vi "insert_spirals.vi"(8 "error in (no error)":errorcluster, 9 "angular shift":dbl, 10 "SpaceVector in":refnum<class "SpaceVector.lvclass">, 11 "TrajectoryDL121017Hopping in":refnum<class "TrajectoryDL121017Hopping.lvclass">) -> (0 "error out":errorcluster, 2 "fix point with spirals":refnum<class "SpaceVector.lvclass">[](array[class]), 3 "TrajectoryDL121017Hopping out":refnum<class "TrajectoryDL121017Hopping.lvclass">)   [LabVIEW 2010, in "TrajectoryDL121017Hopping.lvclass"]
uses:
  TrajectoryDL121017Hopping.lvclass
  common/classes/SpaceVector/SpaceVector/SpaceVector.lvclass
  <vilib>/Native 3D Graph/xcontrol/3DPC_SurfacePlot.xctl
  TrajectoryDL121017Hopping.lvclass/TrajectoryDL121017Hopping.ctl
panel:
  out "3D Graph 2":refnum<class "Base Datatype.lvclass">[](xcontrol)
  in  "number of points":i32=100
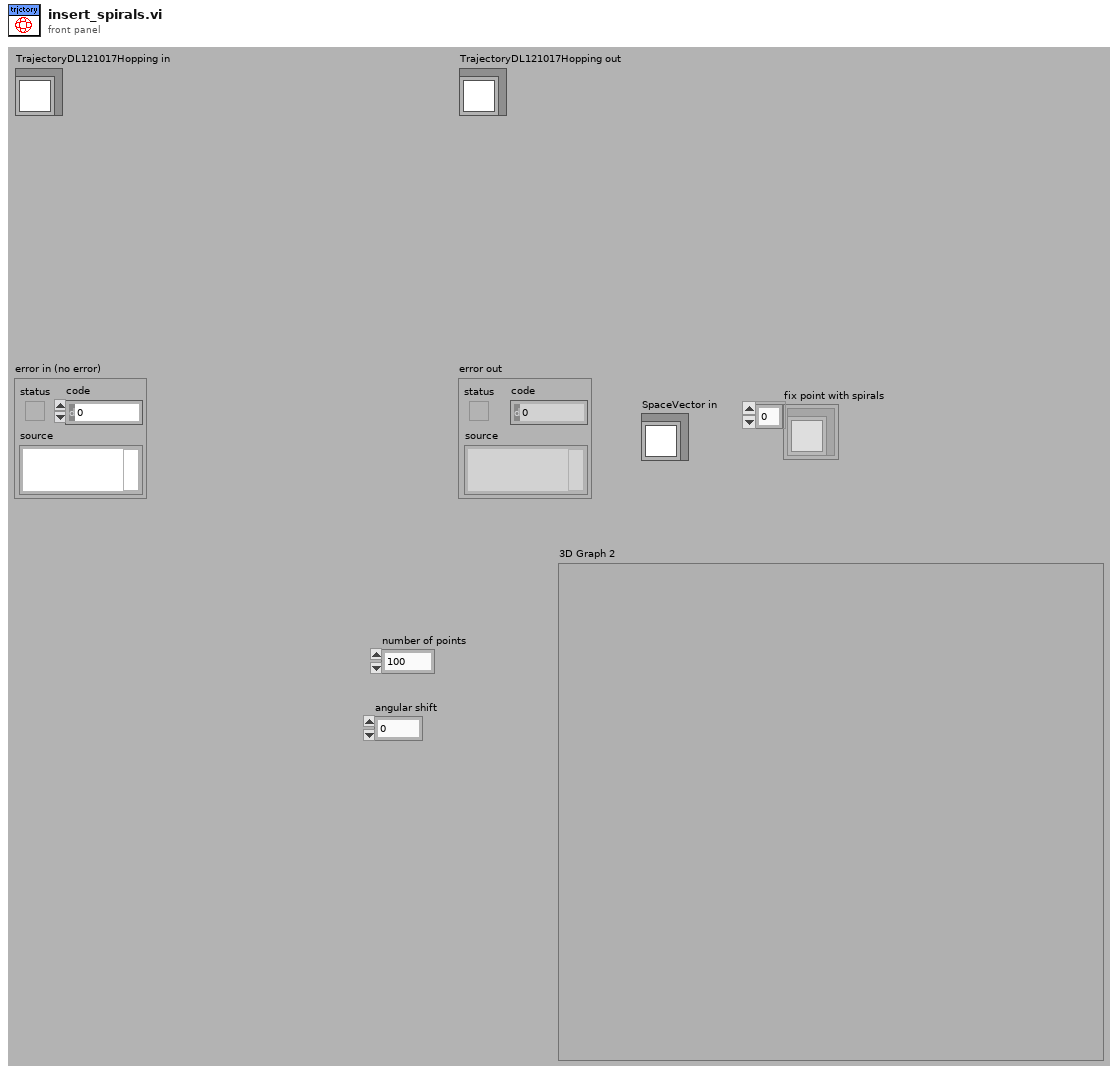
[diagram p1: front panel]
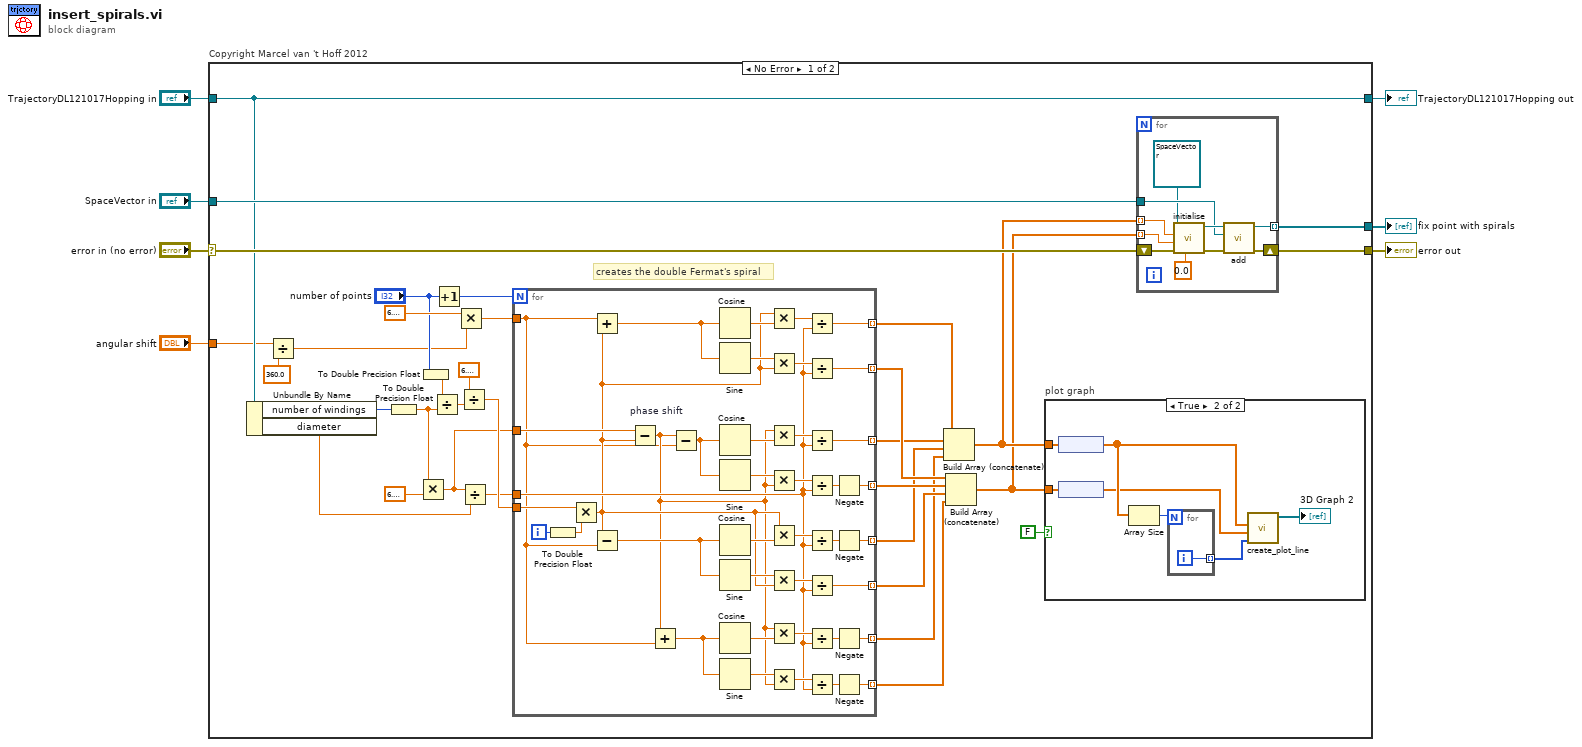
[diagram p0: block diagram]
diagram:
  n1 = case "Copyright Marcel van 't Hoff 2012" shown="No Error" "error in (no error)" {
    selector: "error in (no error)" -> [w36 w100]
    tunnel: [w35 w100] -> w6
    tunnel: [w17 w99] -> w4
    tunnel: "TrajectoryDL121017Hopping in" -> [w17 w99]
    tunnel: [w34 _] -> w3
    tunnel: "SpaceVector in" -> [w32 _]
    tunnel: "angular shift" -> [w13 _]
    frame No Error {
      # "creates the double Fermat's spiral"
      n2 = Unbundle By Name(w17) -> ("number of windings"=w8:i32, "diameter"=w9:dbl[unit])
      n3 = Divide(x=w13, y=360.0) -> (x/y=w11:dbl)
      n4 = To Double Precision Float(number=w8) -> (double precision float=w16:dbl)
      n5 = Multiply(x=w16, y=6.283185307179586) -> (x*y=w25:dbl)
      n6 = To Double Precision Float(number="number of points") -> (double precision float=w38:dbl)
      n7 = Divide(x=w38, y=w16) -> (x/y=w37:dbl)
      n8 = Increment(x="number of points") -> (x+1=w30:i32)
      n9 = Multiply(x=6.283185307179586, y=w11) -> (x*y=w22:dbl)
      n10 = Divide(x=6.283185307179586, y=w37) -> (x/y=w29:dbl)
      n11 = Divide(x=w25, y=w9) -> (x/y=w28:dbl[unit])
      n12 = for {
        N: w30 -> [_]
        tunnel: w29 -> [w88]
        tunnel: [w72] -> w24 mode=indexing
        tunnel: [w81] -> w27 mode=indexing
        tunnel: w28 -> [w60]
        tunnel: w22 -> [w49]
        tunnel: [w74] -> w23 mode=indexing
        tunnel: [w73] -> w26 mode=indexing
        tunnel: w25 -> [w75]
        tunnel: [w65] -> w21 mode=indexing
        tunnel: [w67] -> w20 mode=indexing
        tunnel: [w55] -> w19 mode=indexing
        tunnel: [w54] -> w18 mode=indexing
        i -> [w82]
        n13 = To Double Precision Float(number=w82) -> (double precision float=w83:dbl)
        n14 = Multiply(x=w88, y=w83) -> (x*y=w58:dbl)
        n15 = Add ("add rotation")(x=w49, y=w58) -> (x+y=w53:dbl)
        n16 = Subtract(x=w58, y=w49) -> (x-y=w59:dbl)
        n17 = Subtract "phase shift"(x=w75, y=w58) -> (x-y=w51:dbl)
        n18 = Add(x=w51, y=w49) -> (x+y=w50:dbl)
        n19 = Subtract(x=w51, y=w49) -> (x-y=w52:dbl)
        n20 = Cosine(x=w53) -> (cos(x)=w87:dbl)
        n21 = Sine(x=w53) -> (sin(x)=w86:dbl)
        n22 = Cosine(x=w52) -> (cos(x)=w77:dbl)
        n23 = Sine(x=w52) -> (sin(x)=w78:dbl)
        n24 = Cosine(x=w59) -> (cos(x)=w68:dbl)
        n25 = Sine(x=w59) -> (sin(x)=w69:dbl)
        n26 = Cosine(x=w50) -> (cos(x)=w64:dbl)
        n27 = Sine(x=w50) -> (sin(x)=w63:dbl)
        n28 = Multiply(x=w58, y=w87) -> (x*y=w84:dbl)
        n29 = Multiply(x=w86, y=w58) -> (x*y=w85:dbl)
        n30 = Multiply(x=w51, y=w77) -> (x*y=w80:dbl)
        n31 = Multiply(x=w78, y=w51) -> (x*y=w79:dbl)
        n32 = Multiply(x=w58, y=w68) -> (x*y=w71:dbl)
        n33 = Multiply(x=w69, y=w58) -> (x*y=w70:dbl)
        n34 = Multiply(x=w51, y=w64) -> (x*y=w61:dbl)
        n35 = Multiply(x=w63, y=w51) -> (x*y=w62:dbl)
        n36 = Divide(x=w84, y=w60) -> (x/y=w72:dbl[unit])
        n37 = Divide(x=w85, y=w60) -> (x/y=w81:dbl[unit])
        n38 = Divide(x=w80, y=w60) -> (x/y=w74:dbl[unit])
        n39 = Divide(x=w79, y=w60) -> (x/y=w76:dbl[unit])
        n40 = Divide(x=w71, y=w60) -> (x/y=w66:dbl[unit])
        n41 = Divide(x=w70, y=w60) -> (x/y=w67:dbl[unit])
        n42 = Divide(x=w61, y=w60) -> (x/y=w57:dbl[unit])
        n43 = Divide(x=w62, y=w60) -> (x/y=w56:dbl[unit])
        n44 = Negate(x=w76) -> (-x=w73:dbl[unit])
        n45 = Negate(x=w66) -> (-x=w65:dbl[unit])
        n46 = Negate(x=w57) -> (-x=w55:dbl[unit])
        n47 = Negate(x=w56) -> (-x=w54:dbl[unit])
      }
      n48 = Build Array (concatenate)(w24, w23, w21, w19) -> (w15:dbl[unit][])
      n49 = Build Array (concatenate)(w27, w26, w20, w18) -> (w14:dbl[unit][])
      n50 = case "plot graph" shown="True" FALSE {
        tunnel: w15 -> [_ w47]
        tunnel: w14 -> [_ w46]
        frame False {
        }
        frame True {
          n51 = node(w47) -> (w42:dbl[])
          n52 = node(w46) -> (w41:dbl[])
          n53 = Array Size(array=w42) -> (size(s)=w44:i32)
          n54 = for {
            N: w44 -> [_]
            tunnel: [w48] -> w45 mode=indexing
            i -> [w48]
          }
          n55 = call <vilib>:"create_plot_line.vi"("z vector"=w45, "y vector"=w41, "x vector"=w42) -> ("plots out"=→"3D Graph 2":refnum<class "Base Datatype.lvclass">[])  [unwired: 2 in, 6 out]
        }
      }
      n56 = for {
        tunnel: w32 -> [w93]
        tunnel: w15 -> [w97] mode=indexing
        tunnel: w14 -> [w96] mode=indexing
        shift-right: [w90] -> w35
        shift-left: w36 -> [w98]
        tunnel: [w91] -> w34 mode=indexing
        n57 = call "initialise.vi"("z"=dbl[unit] 0.0, "error in (no error)"=w98, "y"=w96, "x"=w97, "SpaceVector in"=refnum<class "SpaceVector.lvclass"> refnum) -> ("error out"=w95:errorcluster, "SpaceVector out"=w94:refnum<class "SpaceVector.lvclass">)  [unwired: 5 in]
        n58 = call "add.vi"("error in (no error)"=w95, "vector to be added"=w93, "SpaceVector in"=w94) -> ("error out"=w90:errorcluster, "SpaceVector out"=w91:refnum<class "SpaceVector.lvclass">)  [unwired: 7 in]
      }
    }
    frame Error {
    }
  }
  "error out" <- w6
  "TrajectoryDL121017Hopping out" <- w4
  "fix point with spirals" <- w3
